vi "DAQ.Sampling.Find Integer Period Fs and Ns.vi"(9 "f in":dbl, 10 "maxFs":dbl, 11 "sampling in":T1={"Fs"=204789.0, "#s"=15753} {"Fs" format="%#_13g"}) -> (2 "f out":dbl, 3 "sampling out":T1={"Fs"=204789.0, "#s"=15753} {"Fs" format="%#_13g"})   [LabVIEW 2019, in "DAQmx.lvclass"]
uses:
  DAQmx.lvclass
  typedefs/DAQ.Config.Timing.Sampling--Cluster.ctl
panel:
  out "Numeric":i32
  in  "stop":bool
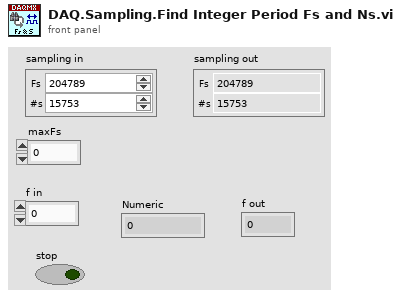
[diagram p1: front panel]
types:
  T1 = typedef "DAQmx.lvclass/DAQ.Config.Timing.Sampling--Cluster.ctl" = cluster{"Fs":dbl, "#s":i32}
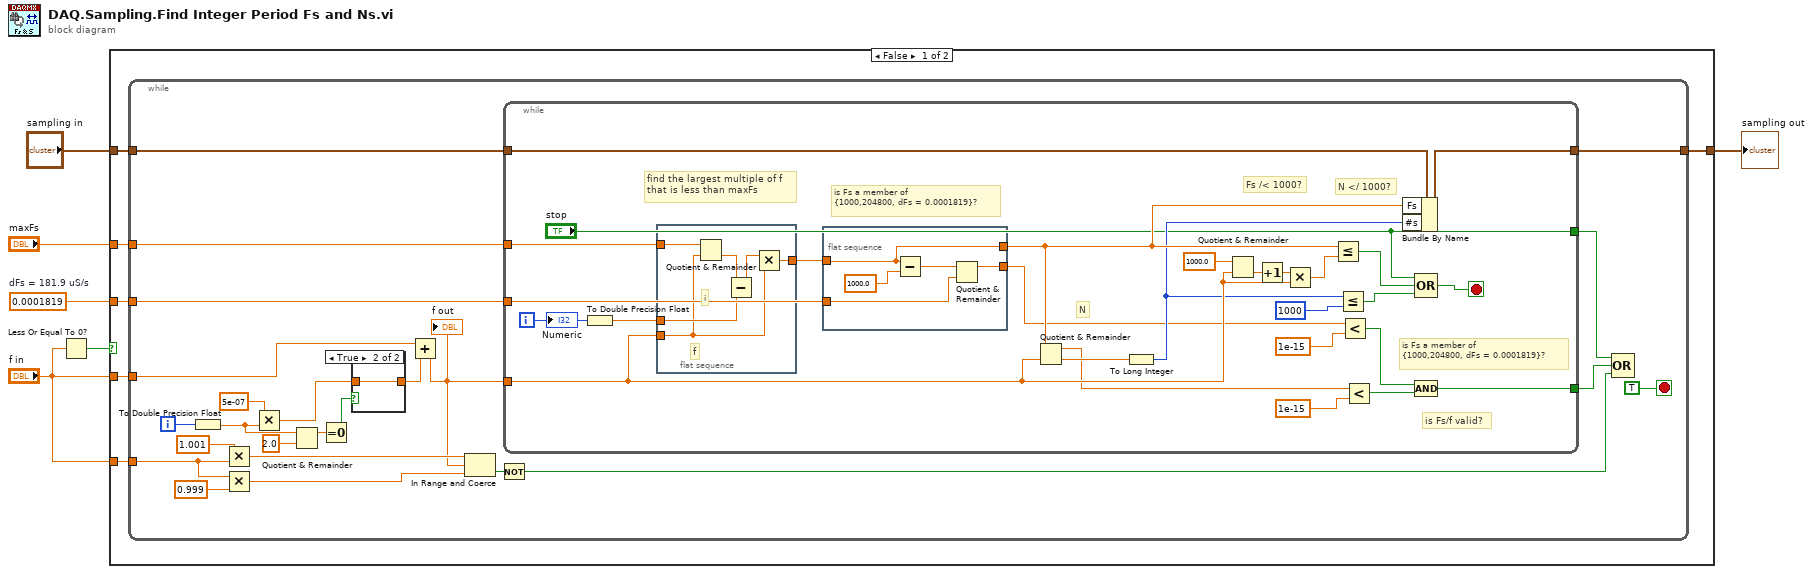
[diagram p0: block diagram]
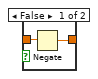
[diagram p2: hidden frame]
diagram:
  w5 = 0.0001819  # dFs = 181.9 uS/s
  n1 = Less Or Equal To 0?(x="f in") -> (x <= 0?=w3:bool)
  n2 = case shown="False" w3 {
    tunnel: "maxFs" -> [w12 _]
    tunnel: "sampling in" -> [w11 w78]
    tunnel: w5 -> [w10 _]
    tunnel: "f in" -> [w9 _]
    tunnel: [w8 w78] -> w2
    tunnel: "f in" -> [w7 _]
    frame False {
      n3 = while {
        tunnel: w12 -> [w36]
        tunnel: w11 -> [w35]
        tunnel: w10 -> [w34]
        tunnel: w9 -> [w32]
        tunnel: [w29] -> w8
        tunnel: w7 -> [w25]
        i -> [w28]
        stop <- TRUE stop-if-true
        n4 = To Double Precision Float(number=w28) -> (double precision float=w20:dbl)
        n5 = Multiply(x=1.001, y=w25) -> (x*y=w26:dbl)
        n6 = Multiply(x=w25, y=0.999 ("x")) -> (x*y=w23:dbl)
        n7 = Multiply(x=5e-07, y=w20) -> (x*y=w15:dbl)
        n8 = Quotient & Remainder(x=w20, y=2.0) -> (x-y*floor(x/y)=w18:dbl)  [unwired: 1 out]
        n9 = Equal To 0?(x=w18) -> (x = 0?=w17:bool)
        n10 = case shown="True" w17 {
          tunnel: [w37 w39] -> w16
          tunnel: w15 -> [w38 w39]
          frame False {
            n11 = Negate(x=w38) -> (-x=w37:dbl)
          }
          frame True {
          }
        }
        n12 = Add(x=w32, y=w16) -> (x+y=w13:dbl)
        "f out" <- w13
        n13 = In Range and Coerce(upper limit=w26, x=w13, lower limit=w23) -> (In Range?=w22:bool)  [unwired: 1 out]
        n14 = Not(x=w22) -> (.not. x?=w21:bool)
        n15 = while {
          tunnel: w36 -> [w66]
          tunnel: w13 -> [w47]
          tunnel: w35 -> [w65]
          tunnel: w34 -> [w64]
          tunnel: [w50] -> w31
          tunnel: ["stop"] -> w30
          tunnel: [w40] -> w29
          i -> [w58]
          stop <- w62 stop-if-true
          # "N </ 1000?"
          # "Fs /< 1000?"
          # "is Fs/f valid?"
          # "is Fs a member of\n{1000,204800, dFs = 0.0001819}?"
          # "N"
          # "is Fs a member of\n{1000,204800, dFs = 0.0001819}?"
          # "find the largest multiple of f\nthat is less than maxFs"
          n16 = To Double Precision Float(number=w58) -> (double precision float=w63:dbl)
          n17 = flat-sequence {
            tunnel: w66 -> [w77]
            tunnel: w63 -> [w76]
            tunnel: w47 -> [w73]
            tunnel: [w72] -> w49
            frame #0 {
              # "i"
              # "f"
              n18 = Quotient & Remainder(x=w77, y=w73) -> (floor(x/y)=w75:dbl)  [unwired: 1 out]
              n19 = Subtract(x=w75, y=w76) -> (x-y=w74:dbl)
              n20 = Multiply(x=w74, y=w73) -> (x*y=w72:dbl)
            }
          }
          n21 = flat-sequence {
            tunnel: [w70] -> w42
            tunnel: w64 -> [w69]
            tunnel: w49 -> [w68]
            tunnel: [w68] -> w60
            frame #0 {
              n22 = Subtract(x=w68, y=1000.0) -> (x-y=w67:dbl)
              n23 = Quotient & Remainder(x=w67, y=w69) -> (x-y*floor(x/y)=w70:dbl)  [unwired: 1 out]
            }
          }
          n24 = Quotient & Remainder(x=w60, y=w47) -> (x-y*floor(x/y)=w46:dbl, floor(x/y)=w54:dbl)
          n25 = To Long Integer(number=w54) -> (32bit integer=w45:i32)
          n26 = Quotient & Remainder(x=1000.0, y=w47) -> (floor(x/y)=w56:dbl)  [unwired: 1 out]
          n27 = Increment(x=w56) -> (x+1=w55:dbl)
          n28 = Multiply(x=w55, y=w47) -> (x*y=w44:dbl)
          n29 = Less Or Equal?(x=w60, y=w44) -> (x <= y?=w59:bool)
          n30 = Less Or Equal?(x=w45, y=1000) -> (x <= y?=w43:bool)
          n31 = Less?(x=w42, y=1e-15 ("upper limit")) -> (x < y?=w48:bool)
          n32 = Less?(x=w46, y=1e-15 ("upper limit")) -> (x < y?=w51:bool)
          n33 = Bundle By Name(cluster=w65, "Fs"=w60, "#s"=w45) -> (w40:T1)
          n34 = Compound Arithmetic op=OR("stop", w59, w43) -> (w62:bool)
          n35 = Compound Arithmetic op=AND(w48, w51) -> (w50:bool)
          "Numeric" <- w58
        }
        n36 = Compound Arithmetic op=OR(w30, w31, w21) -> ()  [unwired: 1 out]
      }
    }
    frame True {
    }
  }
  "sampling out" <- w2
